vi "calcRowAndCols-rgb.vi"(4 "DV":bool, 6 "Ready For Input":bool, 9 "decWidth":u16, 10 "preRow":u16, 11 "preCol":u16) -> (1 "curRow":u16, 3 "curCol":u16)   [LabVIEW 2016]
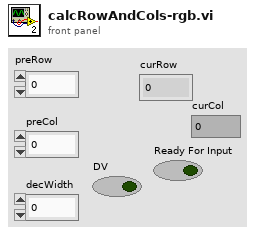
[diagram p1: front panel]
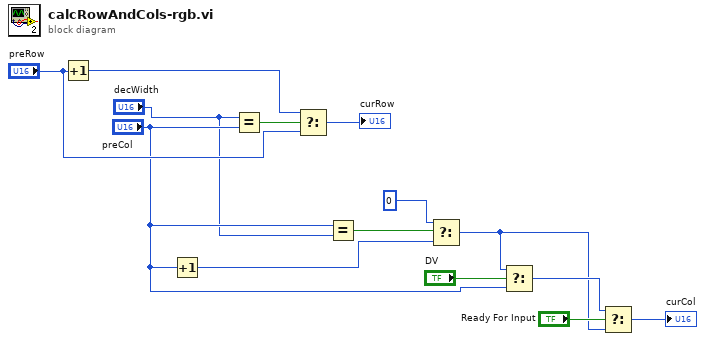
[diagram p0: block diagram]
diagram:
  n1 = Increment(x="preRow") -> (x+1=w13:u16)
  n2 = Increment(x="preCol") -> (x+1=w4:u16)
  n3 = Equal?(x="decWidth", y="preCol") -> (x = y?=w14:bool)
  n4 = Select(t=w13, s=w14, f="preRow") -> (s? t:f=→"curRow":u16)
  n5 = Equal?(x="preCol", y="decWidth") -> (x = y?=w6:bool)
  n6 = Select(t=i16 0, s=w6, f=w4) -> (s? t:f=w3:u16)
  n7 = Select(t=w3, s="DV", f="preCol") -> (s? t:f=w8:u16)
  n8 = Select(t=w8, s="Ready For Input", f=w3) -> (s? t:f=→"curCol":u16)
